vi "Send Image to FPGA (SubVI).vi"(2 "Data Bundle":T5, 3 "Parameters":T1={"File REF"={"AVI REF"=refnum, "DBDE REF"=refnum}, "Frame Data"={"Width"=0, "Height"=0, "Frames Per Second"=0, "Codec"=""}, "File Type"="", "Experiment Mode"=enum."Live", "Movie File Path"=path "D:/Movies Formatted on November 5th 2015/Clip (2) Formatted.raw"}) -> (13 "TimeStamp":u64, 14 "Frame Number":u64, 15 "EOF":bool)   [LabVIEW 2020]
uses:
  Controls (HOST)/REF.ctl
  Controls (HOST)/Image Queue Bundle.ctl
  Controls (HOST)/Data to Disk Bundle.ctl
  Controls (HOST)/File Name Prefix.ctl
  Controls (HOST)/FPGA REF (MWT).ctl
  Controls (HOST)/IMAQ Parameters.ctl
  Controls (HOST)/File REF.ctl
  <vilib>/vision/Avi.llb/IMAQ AVI2 Refnum.ctl
  Controls (HOST)/Experiment Mode.ctl
  <vilib>/Utility/error.llb/Error Cluster From Error Code.vi
  <vilib>/rvi/errors/niLvFpgaAdjustHostInterfaceError.vi
  <vilib>/rvi/interface/nirviMethod/nirviMethod.xnode
  <vilib>/FPGAPlugInAG/Dynamic/niLvFpga_WriteFifo_Dynamic.vi
  <vilib>/rvi/errors/niLvFpgaMergeErrorWithErrorCode.vi
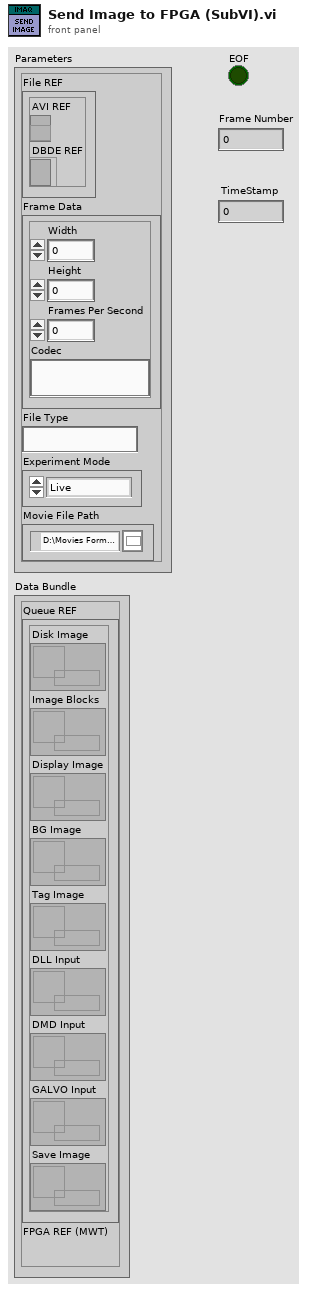
[diagram p1: front panel]
types:
  T1 = typedef "IMAQ Parameters.ctl" = cluster{"File REF":T2, "Frame Data":cluster{"Width":u32, "Height":u32, "Frames Per Second":u32, "Codec":string}, "File Type":string, "Experiment Mode":T4, "Movie File Path":path}
  T2 = typedef "File REF.ctl" = cluster{"AVI REF":T3, "DBDE REF":refnum<file>}
  T3 = typedef "IMAQ AVI2 Refnum.ctl" = refnum<k20>
  T4 = typedef "Experiment Mode.ctl" = enum16{"Live", "Replay"}
  T5 = typedef "REF.ctl" = cluster{"Queue REF":T6, "FPGA REF (MWT)":T7}
  T6 = typedef "Image Queue Bundle.ctl" = cluster{"Disk Image":refnum<queue>, "Image Blocks":refnum<queue>, "Display Image":refnum<queue>, "BG Image":refnum<queue>, "Tag Image":refnum<queue>, "DLL Input":refnum<queue>, "DMD Input":refnum<queue>, "GALVO Input":refnum<queue>, "Save Image":refnum<queue>}
  T7 = typedef "FPGA REF (MWT).ctl" = refnum<k20>
  T8 = enum16{"big-endian, network order", "native, host order", "little-endian"}
  T9 = typedef "IMAQ Image.ctl" = refnum<image>
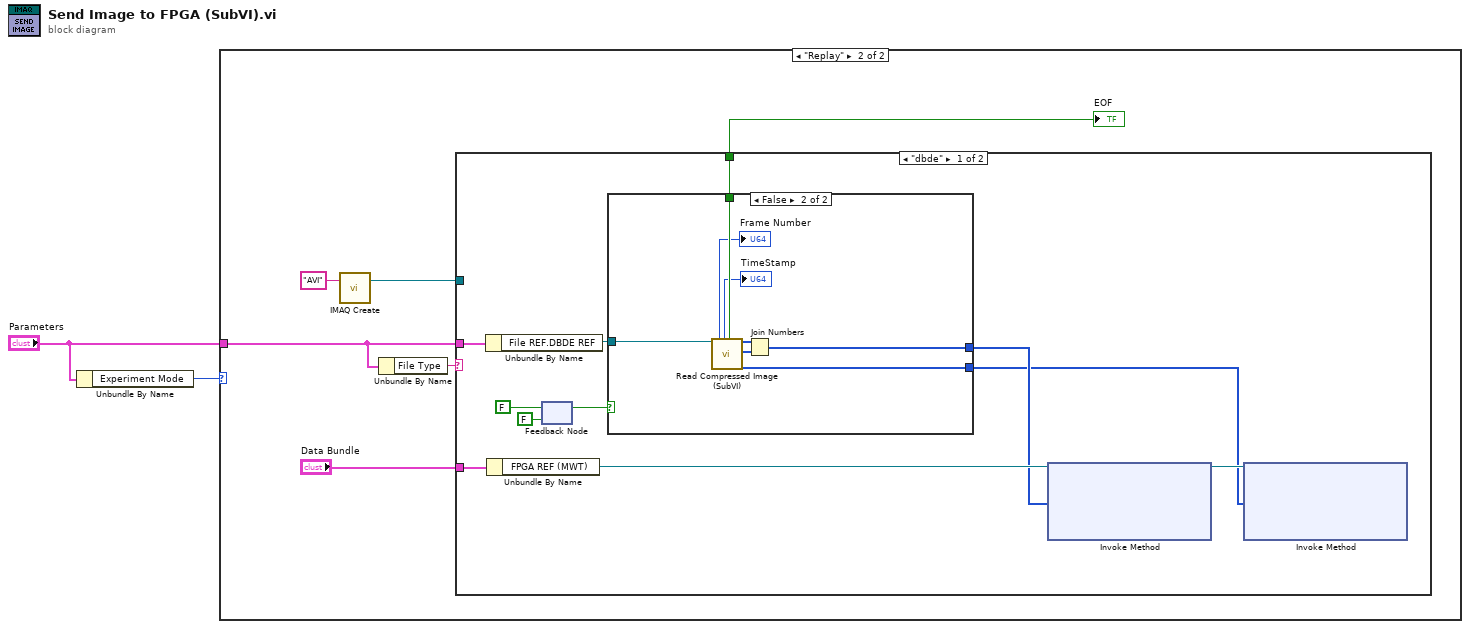
[diagram p0: block diagram]
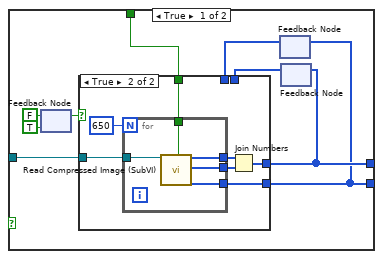
[diagram p3: hidden frame]
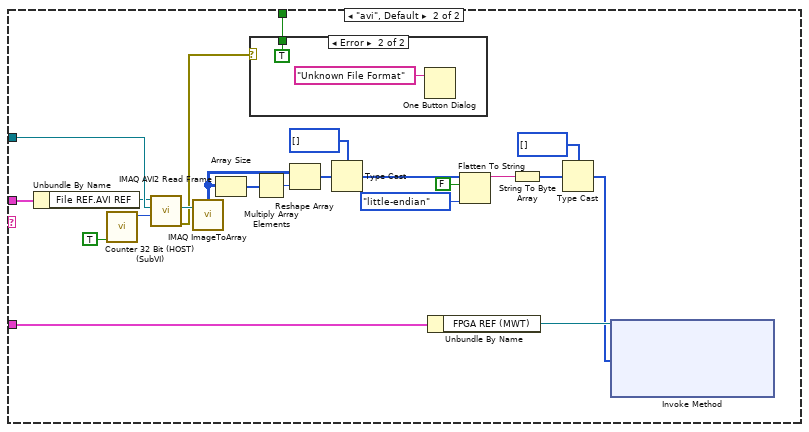
[diagram p5: hidden frame]
diagram:
  n1 = Unbundle By Name("Parameters") -> ("Experiment Mode"=w1:T4)
  n2 = case shown="\"Replay\"" w1 {
    tunnel: "Parameters" -> [_ w4]
    frame "Live", Default {
    }
    frame "Replay" {
      n3 = call "IMAQ Create"("Image Name"="AVI") -> ("New Image"=w8:T9)  [unwired: 4 in, 1 out]
      n4 = Unbundle By Name(w4) -> ("File Type"=w6:string)
      n5 = case shown="\"dbde\"" w6 {
        tunnel: w8 -> [_ w71]
        tunnel: w4 -> [w19 w59]
        tunnel: "Data Bundle" -> [w17 w55]
        tunnel: [w12 w51] -> w3
        frame "dbde" {
          n6 = Unbundle By Name(w19) -> ("File REF.DBDE REF"=w18:refnum<file>)
          n7 = Unbundle By Name(w17) -> ("FPGA REF (MWT)"=w16:T7)
          n8 = feedback-in #1(FALSE) -> ()
          n9 = feedback #1(FALSE) -> (w10:bool)
          n10 = case shown="False" w10 {
            tunnel: w18 -> [w27 w45]
            tunnel: [w22 w49] -> w15
            tunnel: [w21 w47] -> w13
            tunnel: [w28 w46] -> w12
            frame True {
              n11 = feedback-in #2(FALSE) -> ()
              n12 = feedback #2(TRUE) -> (w25:bool)
              n13 = feedback #3() -> (w20:u64[])  [unwired: 1 in]
              n14 = feedback #4() -> (w23:u16[])  [unwired: 1 in]
              n15 = case shown="True" w25 {
                tunnel: [w30 w36] -> w22
                tunnel: [w29 w34] -> w21
                tunnel: [_ w33] -> w28
                tunnel: w27 -> [_ w31]
                tunnel: w23 -> [w30 _]
                tunnel: w20 -> [w29 _]
                frame False {
                }
                frame True {
                  n16 = for {
                    N: 650 -> [_]
                    tunnel: [w42] -> w37
                    tunnel: [w41] -> w35
                    tunnel: [w40] -> w34
                    tunnel: [w39] -> w33
                    tunnel: w31 -> [w38]
                    n17 = call "Read Compressed Image (SubVI).vi"("File REF In"=w38) -> ("EOF"=w39:bool, "Bit Depth"=w42:u8[], "Minimum"=w41:u8[], "Data"=w40:u64[])  [unwired: 13 in, 2 out]
                  }
                  n18 = Join Numbers(hi=w37, lo=w35) -> ((hi.lo)=w36:u16[])
                }
              }
              n19 = feedback-in #3(w21) -> ()
              n20 = feedback-in #4(w22) -> ()
            }
            frame False {
              n21 = call "Read Compressed Image (SubVI).vi"("File REF In"=w45) -> ("Frame Number"=→"Frame Number":u64, "TimeStamp"=→"TimeStamp":u64, "EOF"=w46:bool, "Bit Depth"=w50:u8[], "Minimum"=w48:u8[], "Data"=w47:u64[])  [unwired: 13 in]
              n22 = Join Numbers(hi=w50, lo=w48) -> ((hi.lo)=w49:u16[])
            }
          }
          n23 = xnode "Invoke Method"("FPGA VI Reference In"=w16, "Data"=w15) -> ("FPGA VI Reference Out"=w14:T7)  [unwired: 2 in, 2 out]
          n24 = xnode "Invoke Method"("FPGA VI Reference In"=w14, "Data"=w13) -> ()  [unwired: 2 in, 3 out]
        }
        frame "avi", Default {
          n25 = Unbundle By Name(w59) -> ("File REF.AVI REF"=w58:T3)
          n26 = call "Counter 32 Bit (HOST) (SubVI).vi"("Enable"=TRUE) -> ("Count"=w53:u32)  [unwired: 8 in, 2 out]
          n27 = call "IMAQ AVI2 Read Frame"("Frame Number"=w53, "Image"=w71, "AVI Refnum"=w58) -> ("error out"=w52:errorcluster, "Image Out"=w72:T9)  [unwired: 6 in, 1 out]
          n28 = call "IMAQ ImageToArray"("Image"=w72) -> ("Image Pixels (U8)"=w60:u8[][])  [unwired: 3 in, 4 out]
          n29 = Array Size(array=w60) -> (size(s)=w61:i32[])
          n30 = case shown="Error" w52 {
            tunnel: [_ TRUE ("EOF")] -> w51
            frame No Error {
            }
            frame Error {
              n31 = One Button Dialog(message="Unknown File Format") -> ()  [unwired: 1 in, 1 out]
            }
          }
          n32 = Multiply Array Elements(1:w61) -> (0:w62:i32)
          n33 = Reshape Array(w60, w62) -> (w63:u8[])
          n34 = Type Cast(type=u64[] [], x=w63) -> (*(type *) &x=w65:u64[])
          n35 = Unbundle By Name(w55) -> ("FPGA REF (MWT)"=w57:T7)
          n36 = Flatten To String(anything=w65, prepend array or string size? (T)=FALSE, byte order (0:big-endian, network order)=T8."little-endian") -> (data string=w69:string)  [unwired: 1 in, 2 out]
          n37 = String To Byte Array(string=w69) -> (unsigned byte array=w70:u8[])
          n38 = Type Cast(type=u64[] [], x=w70) -> (*(type *) &x=w56:u64[])
          n39 = xnode "Invoke Method"("FPGA VI Reference In"=w57, "Data"=w56) -> ()  [unwired: 2 in, 3 out]
        }
      }
      "EOF" <- w3
    }
  }
